vi "Calculate Feather Vertices.vi"(6 "2D Feather Property":T3, 8 "error in (no error)":errorcluster, 9 "Base Cluster":T2, 10 "Vertex Cluster":T1, 11 "Plot Area Ref":refnum<vi>) -> (0 "error out":errorcluster, 1 "Feather Vertex":cluster{"X":i16, "Y":i16}[][](array[cluster]), 2 "Center Line Vertex":cluster{"X":i16, "Y":i16}[](array[cluster]), 3 "Dup Plot Area Ref":refnum<vi>)   [LabVIEW 2017, in "2D Feather.lvclass"]
uses:
  <vilib>/Math Plots/2D Math Plots/2D Feather/2D Feather/2D Feather.lvclass
  <vilib>/Math Plots/2D Math Plots/2D Feather/2D Feather/Typedef/2D Feather Property.ctl
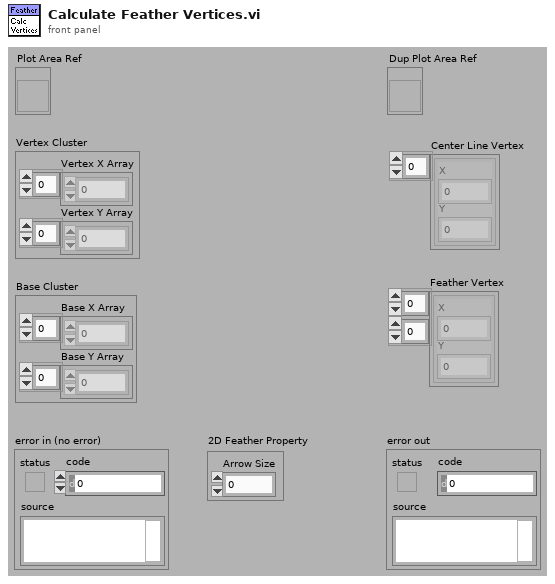
[diagram p1: front panel]
types:
  T1 = cluster{"Vertex X Array":dbl[], "Vertex Y Array":dbl[]}
  T2 = cluster{"Base X Array":dbl[], "Base Y Array":dbl[]}
  T3 = typedef "2D Feather.lvclass/2D Feather Property.ctl" = cluster{"Arrow Size":dbl}
  T4 = typedef "LVPoint32TypeDef.ctl" = cluster{"Horizontal":i32, "Vertical":i32}
  T5 = typedef "LVRectTypeDef.ctl" = cluster{"Left":i16, "Top":i16, "Right":i16, "Bottom":i16}
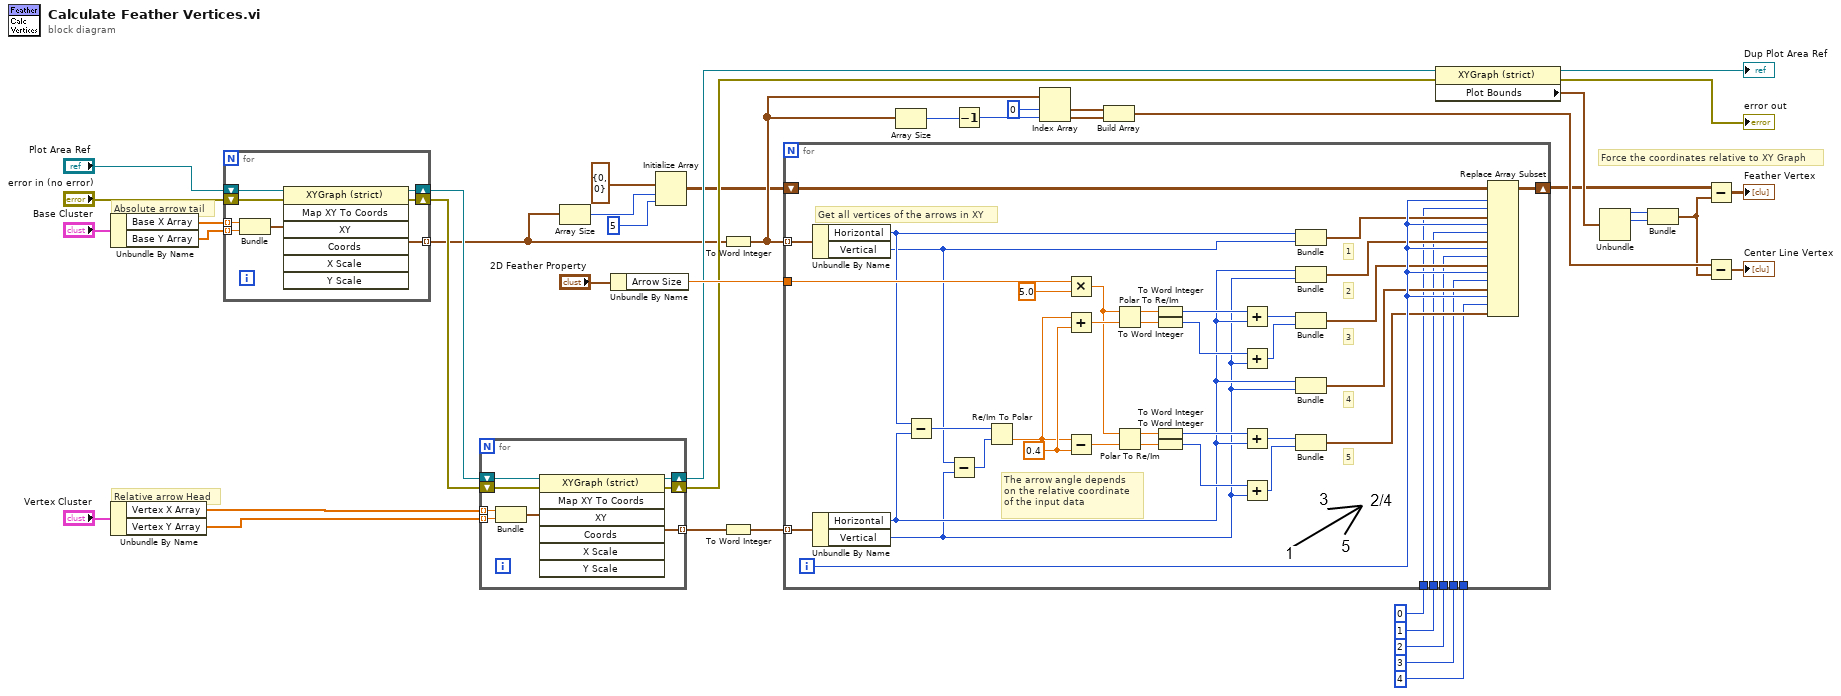
[diagram p0: block diagram]
diagram:
  # "Force the coordinates relative to XY Graph"
  # "Absolute arrow tail"
  # "Relative arrow Head"
  n1 = Unbundle By Name("Base Cluster") -> ("Base X Array"=w15:dbl[], "Base Y Array"=w14:dbl[])
  n2 = Unbundle By Name("Vertex Cluster") -> ("Vertex X Array"=w9:dbl[], "Vertex Y Array"=w13:dbl[])
  n3 = for {
    tunnel: w15 -> [w50] mode=indexing
    tunnel: w14 -> [w49] mode=indexing
    tunnel: [w46] -> w8 mode=indexing
    shift-right: [w45] -> w26
    shift-left: "Plot Area Ref" -> [w47]
    shift-right: [w43] -> w25
    shift-left: "error in (no error)" -> [w44]
    n4 = Bundle("X"=w50, "X"=w49) -> (w48:cluster{"X":dbl, "X":dbl})  [unwired: 1 out]
    n5 = invoke class="XYGraph (strict)" method="Map XY To Coords"(reference=w47, error in=w44, "XY"=w48) -> (reference out=w45:refnum<vi>, error out=w43:errorcluster, "Coords"=w46:T4)  [unwired: 4 in, 4 out]
  }
  n6 = for {
    tunnel: w9 -> [w58] mode=indexing
    tunnel: w13 -> [w57] mode=indexing
    tunnel: [w54] -> w22 mode=indexing
    shift-right: [w53] -> w19
    shift-left: w26 -> [w55]
    shift-right: [w51] -> w18
    shift-left: w25 -> [w52]
    n7 = Bundle("X"=w58, "X"=w57) -> (w56:cluster{"X":dbl, "X":dbl})  [unwired: 1 out]
    n8 = invoke class="XYGraph (strict)" method="Map XY To Coords"(reference=w55, error in=w52, "XY"=w56) -> (reference out=w53:refnum<vi>, error out=w51:errorcluster, "Coords"=w54:T4)  [unwired: 4 in, 4 out]
  }
  n9 = Array Size(array=w8) -> (size(s)=w11:i32)
  n10 = Unbundle By Name("2D Feather Property") -> ("Arrow Size"=w39:dbl)
  n11 = Initialize Array(cluster{"X":i16, "Y":i16} {"X"=0, "Y"=0} ("XY"), w11, 5 ("dimension size")) -> (w7:cluster{"X":i16, "Y":i16}[][])
  n12 = To Word Integer(number=w8) -> (16bit integer=w20:cluster{"Horizontal":i16, "Vertical":i16}[])
  n13 = To Word Integer(number=w22) -> (16bit integer=w21:cluster{"Horizontal":i16, "Vertical":i16}[])
  n14 = for {
    tunnel: w39 -> [w98]
    tunnel: w20 -> [w86] mode=indexing
    tunnel: w21 -> [w87] mode=indexing
    shift-right: [w70] -> w6
    shift-left: w7 -> [w71]
    tunnel: 0 ("disabled index (col)") -> [w63]
    tunnel: 1 ("disabled index (col)") -> [w62]
    tunnel: 2 ("disabled index (col)") -> [w61]
    tunnel: 3 ("disabled index (col)") -> [w60]
    tunnel: 4 ("disabled index (col)") -> [w59]
    i -> [w69]
    w97 = 0.4 ("y")
    # "The arrow angle depends \non the relative coordinate \nof the input data"
    # "Get all vertices of the arrows in XY"
    # "5"
    # "4"
    # "3"
    # "2"
    # "1"
    n15 = Unbundle By Name(w86) -> ("Horizontal"=w77:i16, "Vertical"=w74:i16)
    n16 = Unbundle By Name(w87) -> ("Horizontal"=w78:i16, "Vertical"=w75:i16)
    n17 = Subtract(x=w77, y=w78) -> (x-y=w76:i16)
    n18 = Subtract(x=w74, y=w75) -> (x-y=w73:i16)
    n19 = Re/Im To Polar(2:w73, 3:w76) -> (0:w72:dbl)  [unwired: 1 out]
    n20 = Multiply(x=w98, y=5.0) -> (x*y=w94:dbl)
    n21 = Add(x=w72, y=w97) -> (x+y=w96:dbl)
    n22 = Subtract(x=w72, y=w97) -> (x-y=w95:dbl)
    n23 = Polar To Re/Im(2:w96, 3:w94) -> (0:w92:dbl, 1:w93:dbl)
    n24 = Polar To Re/Im(2:w95, 3:w94) -> (0:w88:dbl, 1:w89:dbl)
    n25 = To Word Integer(number=w93) -> (16bit integer=w83:i16)
    n26 = To Word Integer(number=w92) -> (16bit integer=w81:i16)
    n27 = To Word Integer(number=w89) -> (16bit integer=w85:i16)
    n28 = To Word Integer(number=w88) -> (16bit integer=w84:i16)
    n29 = Add(x=w83, y=w78) -> (x+y=w82:i16)
    n30 = Add(x=w81, y=w75) -> (x+y=w80:i16)
    n31 = Add(x=w85, y=w78) -> (x+y=w91:i16)
    n32 = Add(x=w84, y=w75) -> (x+y=w90:i16)
    n33 = Bundle("Horizontal"=w77, "Vertical"=w74) -> (w68:cluster{"Horizontal":i16, "Vertical":i16})  [unwired: 1 out]
    n34 = Bundle("Horizontal"=w78, "Vertical"=w75) -> (w67:cluster{"Horizontal":i16, "Vertical":i16})  [unwired: 1 out]
    n35 = Bundle(w82, w80) -> (w66:cluster{i16, i16})  [unwired: 1 out]
    n36 = Bundle("Horizontal"=w78, "Vertical"=w75) -> (w65:cluster{"Horizontal":i16, "Vertical":i16})  [unwired: 1 out]
    n37 = Bundle(w91, w90) -> (w64:cluster{i16, i16})  [unwired: 1 out]
    n38 = Replace Array Subset(array=w71, new element #1=w68, index (row) #1=w69, index (col) #1=w63, new element #2=w67, index (row) #2=w69, index (col) #2=w62, new element #3=w66, index (row) #3=w69, index (col) #3=w61, new element #4=w65, index (row) #4=w69, index (col) #4=w60, new element #5=w64, index (row) #5=w69, index (col) #5=w59) -> (w70:cluster{"X":i16, "Y":i16}[][])
  }
  n39 = Array Size(array=w20) -> (size(s)=w32:i32)
  n40 = Decrement(x=w32) -> (x-1=w31:i32)
  n41 = Index Array(array=w20, index #1=0 ("index"), index #2=w31) -> (element #1=w17:cluster{"Horizontal":i16, "Vertical":i16}, element #2=w16:cluster{"Horizontal":i16, "Vertical":i16})
  n42 = Build Array(w17, w16) -> (w29:cluster{"Horizontal":i16, "Vertical":i16}[])
  n43 = property class="XYGraph (strict)"(reference=w19, error in=w18) -> (reference out=→"Dup Plot Area Ref":refnum<vi>, error out=→"error out":errorcluster, "Plot Bounds"=w37:T5)
  n44 = Unbundle(w37) -> ("Left"=w35:i16, "Top"=w36:i16)  [unwired: 2 out]
  n45 = Bundle("Left"=w35, "Top"=w36) -> (w28:cluster{"Left":i16, "Top":i16})  [unwired: 1 out]
  n46 = Subtract(x=w6, y=w28) -> (x-y=→"Feather Vertex":cluster{i16, i16}[][])
  n47 = Subtract(x=w29, y=w28) -> (x-y=→"Center Line Vertex":cluster{i16, i16}[])
